vi "Test vibratome3.vi"() -> ()   [LabVIEW 2018]
uses:
  General/Controls/Translation Stage Parameters.ctl
  Hardware Mfg/Thorlabs Translation Stages/Controls/Translation Stage Cluster.ctl
  General/Controls/Translation Stage Types.ctl
  Hardware Mfg/Thorlabs Translation Stages/Controls/Motion Translation Module Control2.ctl
  General/Controls/Set Get Controls.ctl
panel:
  in  "Table Stages":T1={"X Stage"={"Position"=25.0, "Is.Enabled?"=FALSE, "Is.Connected?"=FALSE, "Device SN"="45876425", "AccelerationMaximum"=10.0, "VelocityMaximum"=10.0, "Acceleration"=10.0, "Velocity"=10.0, "waitTimeout (ms)"=1111110, "Model"=enum."Thorlabs LTS", "Is.Homed?"=FALSE}, "Y Stage"={"Position"=89.0, "Is.Enabled?"=FALSE, "Is.Connected?"=FALSE, "Device SN"="45995820", "AccelerationMaximum"=10.0, "VelocityMaximum"=10.0, "Acceleration"=10.0, "Velocity"=10.0, "waitTimeout (ms)"=1111110, "Model"=enum."Thorlabs LTS", "Is.Homed?"=FALSE}, "Z Stage"={"Position"=0.0, "Is.Enabled?"=FALSE, "Is.Connected?"=FALSE, "Device SN"="45876539", "AccelerationMaximum"=0.0, "VelocityMaximum"=0.0, "Acceleration"=0.0, "Velocity"=0.0, "waitTimeout (ms)"=0, "Model"=enum."None", "Is.Homed?"=FALSE}}
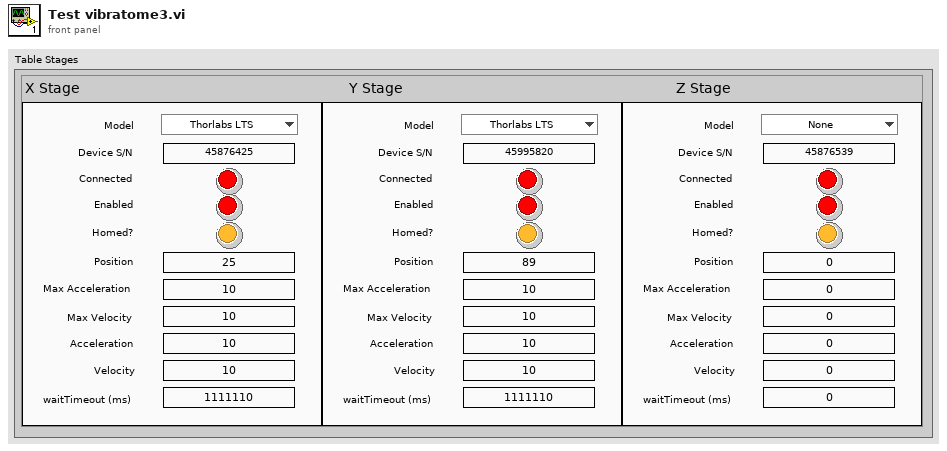
[diagram p1: front panel]
types:
  T1 = typedef "Translation Stage Parameters.ctl" = cluster{"X Stage":T2, "Y Stage":T2, "Z Stage":T2}
  T2 = typedef "Translation Stage Cluster.ctl" = cluster{"Position":dbl, "Is.Enabled?":bool, "Is.Connected?":bool, "Device SN":string, "AccelerationMaximum":dbl, "VelocityMaximum":dbl, "Acceleration":dbl, "Velocity":dbl, "waitTimeout (ms)":i32, "Model":T3, "Is.Homed?":bool}
  T3 = typedef "Translation Stage Types.ctl" = enum16{"None", "Thorlabs LTS", "Thorlabs MLJ"}
  T4 = typedef "Set Get Controls.ctl" = enum16{"Set", "Get"}
  T5 = typedef "Motion Translation Module Control2.ctl" = enum16{"Init", "Home", "Status", "Velocity/Accel", "Position", "Jog", "Stop", "Uninit", "Enable", "Disable"}
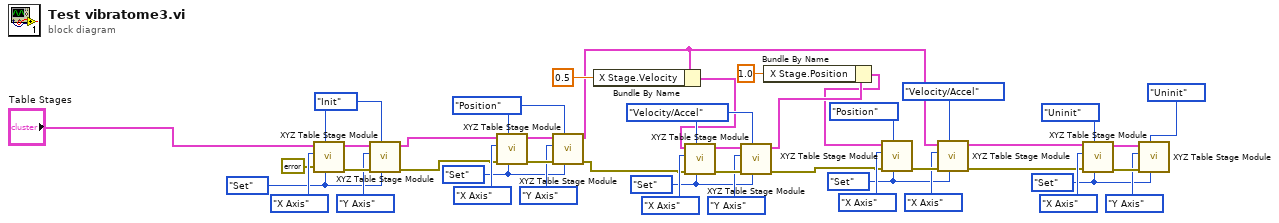
[diagram p0: block diagram]
diagram:
  w1 = Set_Get_Controls."Set" ("Set/Get")
  w20 = Set_Get_Controls."Set" ("Set/Get")
  w27 = Set_Get_Controls."Set" ("Set/Get")
  w26 = Motion_Translation_Module_Control2."Velocity/Accel" ("Action")
  w36 = Set_Get_Controls."Set" ("Set/Get")
  w35 = Motion_Translation_Module_Control2."Position" ("Action")
  w42 = Set_Get_Controls."Set" ("Set/Get")
  w41 = Motion_Translation_Module_Control2."Init" ("Action")
  n1 = call "XYZ Table Stage Module.vi"("Set/Get"=w42, "Action"=w41, "Error In"=errorcluster {"status"=FALSE, "code"=0, "source"=""}, "Axis"=enum16{"X Axis", "Y Axis", "Z Axis"}."X Axis", "Table Stages"="Table Stages") -> ("Error Out"=w45:errorcluster, "Table Stages [out]"=w33:T1)  [unwired: 5 in]
  n2 = call "XYZ Table Stage Module.vi"("Set/Get"=w42, "Action"=w41, "Error In"=w45, "Axis"=enum16{"X Axis", "Y Axis", "Z Axis"}."Y Axis", "Table Stages"=w33) -> ("Error Out"=w34:errorcluster, "Table Stages [out]"=w32:T1)  [unwired: 5 in]
  n3 = call "XYZ Table Stage Module.vi"("Set/Get"=w36, "Action"=w35, "Error In"=w34, "Axis"=enum16{"X Axis", "Y Axis", "Z Axis"}."X Axis", "Table Stages"=w32) -> ("Error Out"=w39:errorcluster, "Table Stages [out]"=w31:T1)  [unwired: 5 in]
  n4 = call "XYZ Table Stage Module.vi"("Set/Get"=w36, "Action"=w35, "Error In"=w39, "Axis"=enum16{"X Axis", "Y Axis", "Z Axis"}."Y Axis", "Table Stages"=w31) -> ("Error Out"=w24:errorcluster, "Table Stages [out]"=w11:T1)  [unwired: 5 in]
  n5 = Bundle By Name(cluster=w11, "X Stage.Velocity"=0.5) -> (w14:T1)
  n6 = call "XYZ Table Stage Module.vi"("Set/Get"=w27, "Action"=w26, "Error In"=w24, "Axis"=enum16{"X Axis", "Y Axis", "Z Axis"}."X Axis", "Table Stages"=w14) -> ("Error Out"=w30:errorcluster, "Table Stages [out]"=w25:T1)  [unwired: 5 in]
  n7 = call "XYZ Table Stage Module.vi"("Set/Get"=w27, "Action"=w26, "Error In"=w30, "Axis"=enum16{"X Axis", "Y Axis", "Z Axis"}."Y Axis", "Table Stages"=w25) -> ("Error Out"=w18:errorcluster, "Table Stages [out]"=w13:T1)  [unwired: 5 in]
  n8 = Bundle By Name(cluster=w13, "X Stage.Position"=1.0) -> (w12:T1)
  n9 = call "XYZ Table Stage Module.vi"("Set/Get"=w20, "Action"=Motion_Translation_Module_Control2."Position", "Error In"=w18, "Axis"=enum16{"X Axis", "Y Axis", "Z Axis"}."X Axis", "Table Stages"=w12) -> ("Error Out"=w23:errorcluster)  [unwired: 5 in, 1 out]
  n10 = call "XYZ Table Stage Module.vi"("Set/Get"=w20, "Action"=Motion_Translation_Module_Control2."Velocity/Accel", "Error In"=w23, "Axis"=enum16{"X Axis", "Y Axis", "Z Axis"}."X Axis", "Table Stages"=w11) -> ("Error Out"=w5:errorcluster, "Table Stages [out]"=w4:T1)  [unwired: 5 in]
  n11 = call "XYZ Table Stage Module.vi"("Set/Get"=w1, "Action"=Motion_Translation_Module_Control2."Uninit", "Error In"=w5, "Axis"=enum16{"X Axis", "Y Axis", "Z Axis"}."X Axis", "Table Stages"=w4) -> ("Error Out"=w9:errorcluster, "Table Stages [out]"=w3:T1)  [unwired: 5 in]
  n12 = call "XYZ Table Stage Module.vi"("Set/Get"=w1, "Action"=Motion_Translation_Module_Control2."Uninit", "Error In"=w9, "Axis"=enum16{"X Axis", "Y Axis", "Z Axis"}."Y Axis", "Table Stages"=w3) -> ()  [unwired: 5 in, 2 out]
